vi "QueryChannelSettings.vi"(8 "error in":errorcluster, 11 "T560Session in":refnum<class "T560Session.lvclass">) -> (0 "error out":errorcluster, 3 "T560Session out":refnum<class "T560Session.lvclass">)   [LabVIEW 2013, in "Highlandt564.lvlib" / "T560Session.lvclass"]
doc: "Read the channels configuration from the physical device"
uses:
  T560Session.lvclass
  T560Session.lvclass/T560Session.ctl
  T560ChannelClass/T560Channel.lvclass
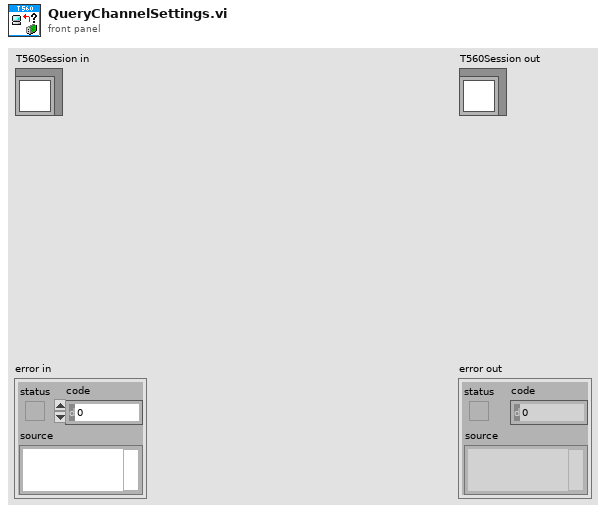
[diagram p1: front panel]
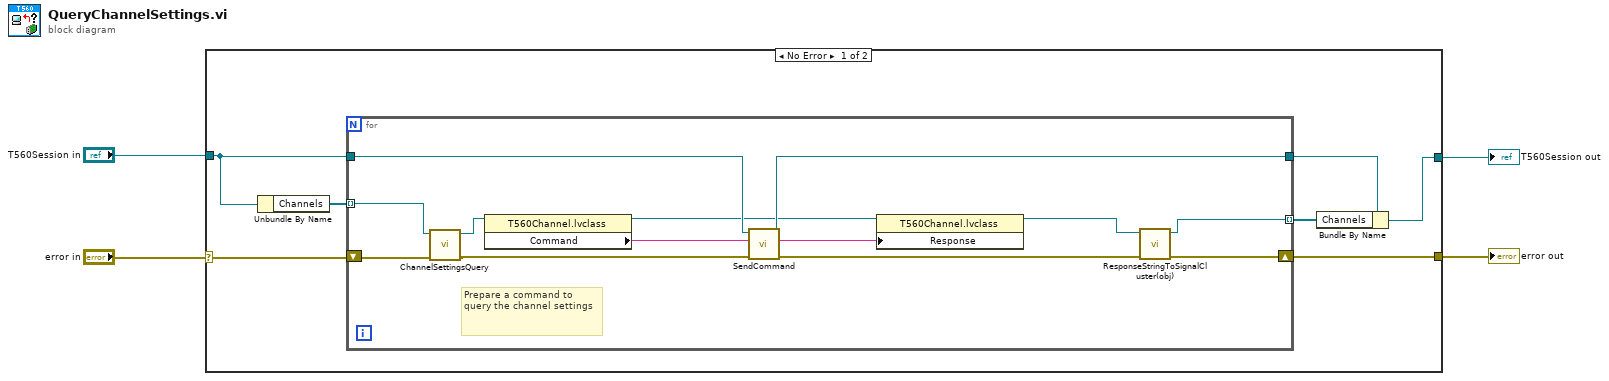
[diagram p0: block diagram]
diagram:
  n1 = case shown="No Error" "error in" {
    selector: "error in" -> [w10 w26]
    tunnel: [w9 w26] -> w3
    tunnel: [w5 w25] -> w1
    tunnel: "T560Session in" -> [w8 w25]
    frame No Error {
      n2 = Unbundle By Name(w8) -> ("Channels"=w11:refnum<class "T560Channel.lvclass">[])
      n3 = for {
        tunnel: w11 -> [w22] mode=indexing
        tunnel: w8 -> [w21]
        shift-right: [w13] -> w9
        shift-left: w10 -> [w24]
        tunnel: [w20] -> w7
        tunnel: [w15] -> w6 mode=indexing
        # "Prepare a command to query the channel settings"
        n4 = call-dynamic "ChannelSettingsQuery.vi"("error in"=w24, "T560Object in"=w22) -> ("error out"=w17:errorcluster, "T560Object out"=w19:refnum<class "T560Channel.lvclass">)  [unwired: 8 in]
        n5 = property class="T560Channel.lvclass"(reference=w19) -> (reference out=w18:refnum<class "T560Channel.lvclass">, "Command"=w23:string)  [unwired: 1 in, 1 out]
        n6 = call-dynamic "SendCommand.vi"("error in"=w17, "Command"=w23, "T560Session in"=w21) -> ("error out"=w14:errorcluster, "Response"=w12:string, "T560Session out"=w20:refnum<class "T560Session.lvclass">)  [unwired: 6 in]
        n7 = property class="T560Channel.lvclass"(reference=w18, "Response"=w12) -> (reference out=w16:refnum<class "T560Channel.lvclass">)  [unwired: 1 in, 1 out]
        n8 = call-dynamic "ResponseStringToSignalCluster(obj).vi"("error in (no error)"=w14, "T560Channel in"=w16) -> ("error out"=w13:errorcluster, "T560Channel out"=w15:refnum<class "T560Channel.lvclass">)  [unwired: 8 in]
      }
      n9 = Bundle By Name(cluster=w7, "Channels"=w6) -> (w5:refnum<class "T560Session.lvclass">)
    }
    frame Error {
    }
  }
  "error out" <- w3
  "T560Session out" <- w1
